vi "Set Port Power.vi"(0 "VISA resource name":refnum<visa-resource-name>, 1 "Channel (1)":i32=1, 2 "Port (1)":i32=1, 5 "Power Level (0.0)":dbl format="%^.3g", 11 "error in (no error)":errorcluster, 12 "Offset":dbl format="%#_13g", 13 "RO(t)":bool) -> (3 "pow level(rd)":dbl format="%.3g", 4 "VISA resource name out":refnum<visa-resource-name>, 15 "error out":errorcluster)   [LabVIEW 2018, in "Agilent ENA Series.lvlib"]
doc: "Configures power settings.\n\n<b>Note:</b>\nThis VI is not supported by the E5063A model."
uses:
  Agilent ENA Series.lvlib
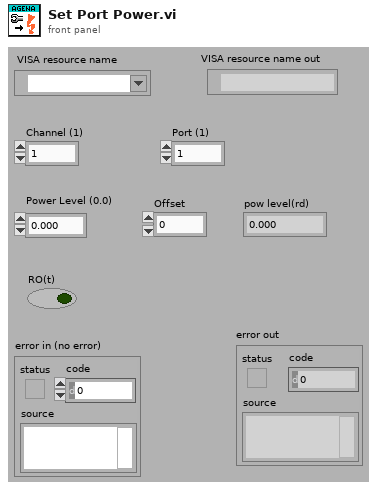
[diagram p1: front panel]
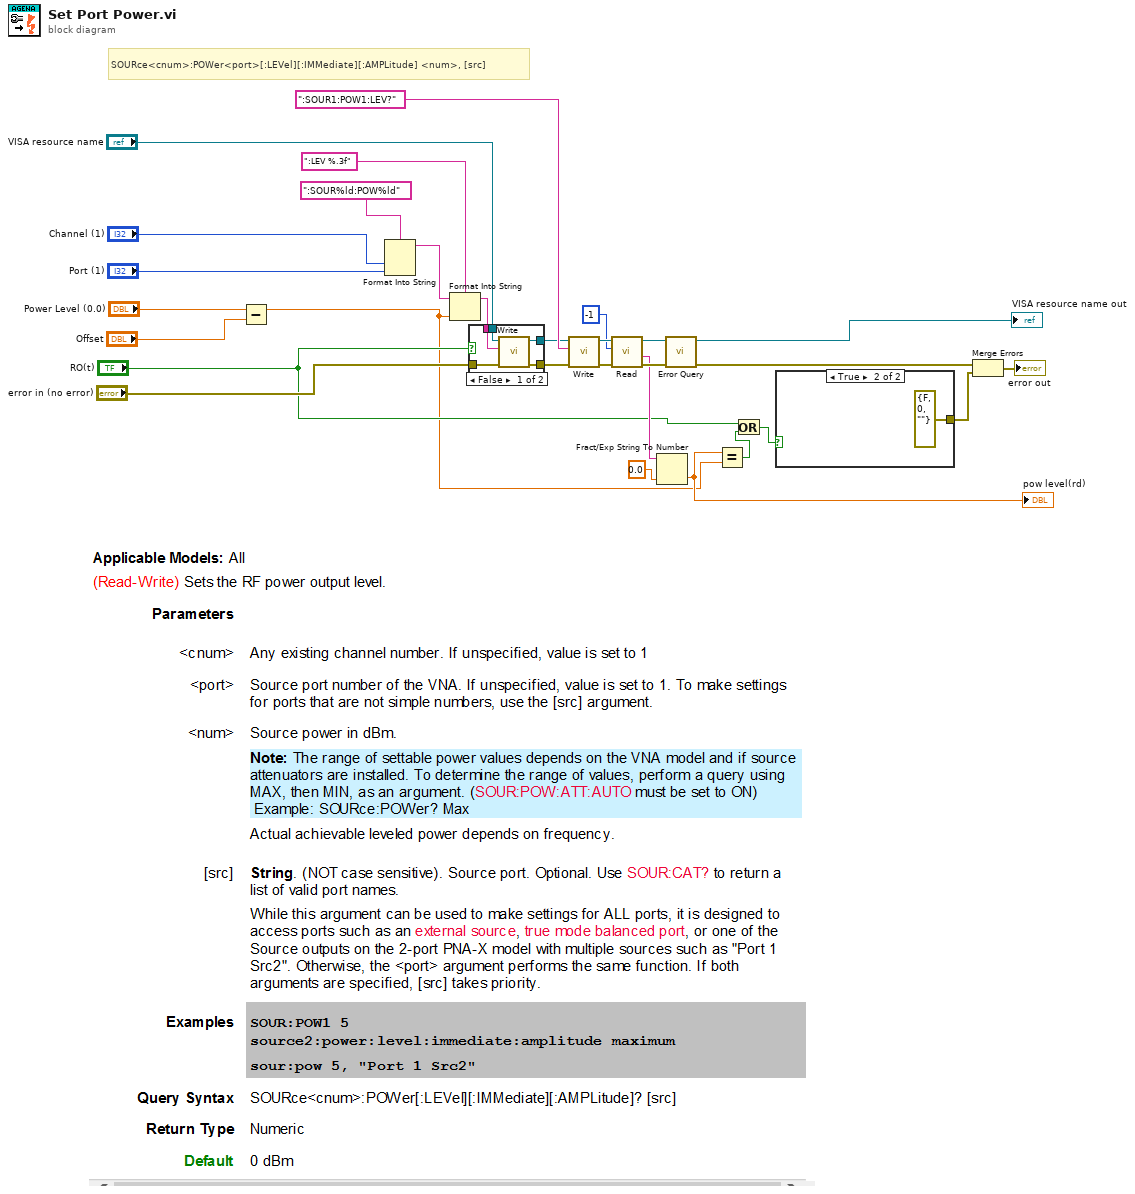
[diagram p0: block diagram]
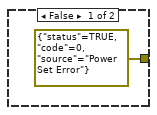
[diagram p3: hidden frame]
diagram:
  # "SOURce<cnum>:POWer<port>[:LEVel][:IMMediate][:AMPLitude] <num>, [src]"
  n1 = Subtract(x="Power Level (0.0)", y="Offset") -> (x-y=w2:dbl)
  n2 = Format Into String(format string=":SOUR%ld:POW%ld", "Channel (1)", "Port (1)") -> (resulting string=w25:string)  [unwired: 2 in, 1 out]
  n3 = Format Into String(format string=":LEV %.3f", initial string=w25, w2) -> (resulting string=w22:string)  [unwired: 1 in, 1 out]
  n4 = case shown="False" "RO(t)" {
    tunnel: "error in (no error)" -> [w34 w35]
    tunnel: w22 -> [w33 _]
    tunnel: "VISA resource name" -> [w32 w36]
    tunnel: [w31 w35] -> w17
    tunnel: [w30 w36] -> w6
    frame False {
      n5 = call "Write.vi"("error in (no error)"=w34, "String ()"=w33, "VISA resource name"=w32) -> ("error out"=w31:errorcluster, "VISA resource name out"=w30:refnum<visa-resource-name>)  [unwired: 6 in, 1 out]
    }
    frame True {
    }
  }
  n6 = call "Write.vi"("error in (no error)"=w17, "String ()"=":SOUR1:POW1:LEV?", "VISA resource name"=w6) -> ("error out"=w19:errorcluster, "VISA resource name out"=w20:refnum<visa-resource-name>)  [unwired: 6 in, 1 out]
  n7 = call "Read.vi"("error in (no error)"=w19, "Number Of Bytes"=-1, "VISA resource name"=w20) -> ("error out"=w16:errorcluster, "String"=w13:string, "VISA resource name out"=w15:refnum<visa-resource-name>)  [unwired: 5 in, 1 out]
  n8 = Fract/Exp String To Number(string=w13, default (0 dbl)=0.0 ("default (0 DBL)")) -> (number=w11:dbl)  [unwired: 2 in, 1 out]
  "pow level(rd)" <- w11
  n9 = call "Error Query.vi"("error in (no error)"=w16, "VISA resource name"=w15) -> ("error out"=w8:errorcluster, "VISA resource name out"=→"VISA resource name out":refnum<visa-resource-name>)  [unwired: 6 in, 2 out]
  n10 = Equal?(x=w11, y=w2) -> (x = y?=w5:bool)
  n11 = Or(x="RO(t)", y=w5) -> (x .or. y?=w4:bool)
  n12 = case shown="True" w4 {
    tunnel: [errorcluster {"status"=TRUE, "code"=0, "source"="Power Set Error"} ("error constant") errorcluster {"status"=FALSE, "code"=0, "source"=""} ("error constant")] -> w9
    frame False {
    }
    frame True {
    }
  }
  n13 = Merge Errors(w8, w9) -> (→"error out":errorcluster)
